vi "Read INI file.vi"(0 "Path":path=path "C:/Users/Priyanka/Documents/Plotter/Data/Plot Configuration.txt", 11 "error in (no error)":errorcluster) -> (3 "Available Devices":string[](array[string]), 4 "Data":string[][](array[string]), 6 "No of variables":string[](array[string]), 8 "Display Names":string[](array[string]), 10 "References":string[](array[string]), 15 "error out":errorcluster)   [LabVIEW 2020]
doc: "This vi reads the configuration file for device variables and parse the data.\n[Inputs]\n1. File input\n2. Error in\n[output]\n1. Data (read from configuration file)\n2. Available Devices\n3. No of variables for devices\n4. References for data plot\n5. variable Display names"
uses:
  <vilib>/Utility/config.llb/Read Key (String).vi
  <userlib>/_OpenG.lib/array/array.llb/Remove Duplicates from 1D Array (String)__ogtk.vi
  <vilib>/Utility/config.llb/NI_LVConfig.lvlib
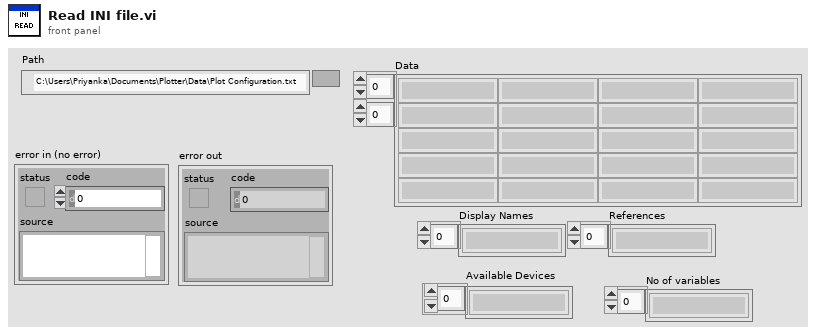
[diagram p1: front panel]
types:
  T1 = typedef "NI_LVConfig.lvlib/Config Data RefNum.ctl" = refnum<k1>
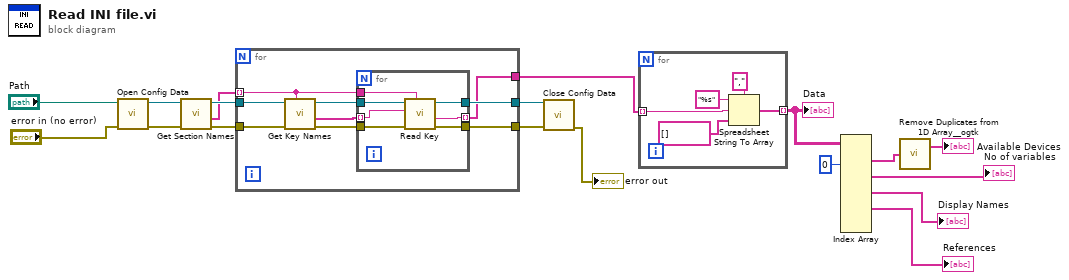
[diagram p0: block diagram]
diagram:
  n1 = call <vilib>:"Open Config Data.vi"("error in (no error)"="error in (no error)", "configuration file path"="Path") -> ("error out"=w16:errorcluster, "refnum"=w15:T1)  [unwired: 7 in, 1 out]
  n2 = call <vilib>:"Get Section Names.vi"("error in (no error)"=w16, "refnum"=w15) -> ("error out"=w13:errorcluster, "section names"=w12:string[], "refnum out"=w14:T1)  [unwired: 7 in]
  n3 = for {
    tunnel: w14 -> [w27]
    tunnel: w13 -> [w26]
    tunnel: w12 -> [w22] mode=indexing
    tunnel: [w21] -> w11
    tunnel: [w20] -> w10
    tunnel: [w19] -> w9
    n4 = call <vilib>:"Get Key Names.vi"("section"=w22, "error in (no error)"=w26, "refnum"=w27) -> ("error out"=w24:errorcluster, "key names"=w23:string[], "refnum out"=w25:T1)  [unwired: 5 in, 1 out]
    n5 = for {
      tunnel: w25 -> [w34]
      tunnel: w24 -> [w33]
      tunnel: w23 -> [w32] mode=indexing
      tunnel: w22 -> [w31]
      tunnel: [w30] -> w21
      tunnel: [w29] -> w20
      tunnel: [w28] -> w19 mode=indexing
      n6 = call-poly <vilib>:"Read Key.vi"("section"=w31, "error in (no error)"=w33, "key"=w32, "refnum"=w34) -> ("error out"=w29:errorcluster, "value"=w28:string, "refnum out"=w30:T1)  [unwired: 4 in, 1 out]
    }
  }
  n7 = call <vilib>:"Close Config Data.vi"("error in (no error)"=w10, "refnum"=w11) -> ("error out"=→"error out":errorcluster)  [unwired: 8 in, 1 out]
  n8 = for {
    tunnel: w9 -> [w37] mode=indexing
    tunnel: [w35] -> w7 mode=indexing
    n9 = Spreadsheet String To Array(delimiter (Tab)=",", format string="%s", spreadsheet string=w37, array type (2D Dbl)=string[] []) -> (array=w35:string[])
  }
  "Data" <- w7
  n10 = Index Array(array=w7, index (col) #1=0 ("disabled index (col)")) -> (element #1=w5:string[], element #2=→"No of variables":string[], element #3=→"Display Names":string[], element #4=→"References":string[])  [unwired: 9 in, 1 out]
  n11 = call-poly <userlib>:"Remove Duplicates from 1D Array__ogtk.vi"("Input Array"=w5) -> ("Output Array"=→"Available Devices":string[])  [unwired: 1 out]
